vi "List Queues.vi"(6 "Name Prefix":string, 8 "error in (no error)":errorcluster, 9 "Region":T1, 11 "AWS Credentials":T2) -> (0 "error out":errorcluster, 3 "SQS Queues":refnum<class "Queue.lvclass">[](array[class]))   [LabVIEW 2015, in "NI_AWS_SQS.lvlib" / "Queue.lvclass"]
doc: "Returns a list of your queues. The maximum number of queues that can be returned is 1,000. If you specify a value for the optional QueueNamePrefix parameter, only queues with a name that begins with the specified value are returned."
uses:
  Queue.lvclass
  Core/HTTP Request/AWS Credentials.ctl
  Core/HTTP Request/Region.ctl
  Core/HTTP Request/Request Options.ctl
  Core/HTTP Request/Name Value Pair.ctl
  Core/HTTP Request/Region handling.ctl
  Core/HTTP Request/URL formatting.ctl
  Core/HTTP Request/HTTP Request.lvclass/HTTP Request.ctl
  Queue.lvclass/Queue.ctl
  Write Account Number.vi
  Write Name.vi
  Write URL.vi
  Core/HTTP Request/Write Credentials.vi
  Core/HTTP Request/Write Region.vi
  Core/HTTP Request/Write Service.vi
  Core/HTTP Request/Write Verify Server.vi
  Core/HTTP Request/HTTP Request.lvclass
  XML Parsing/NI_XML Parsing.lvlib
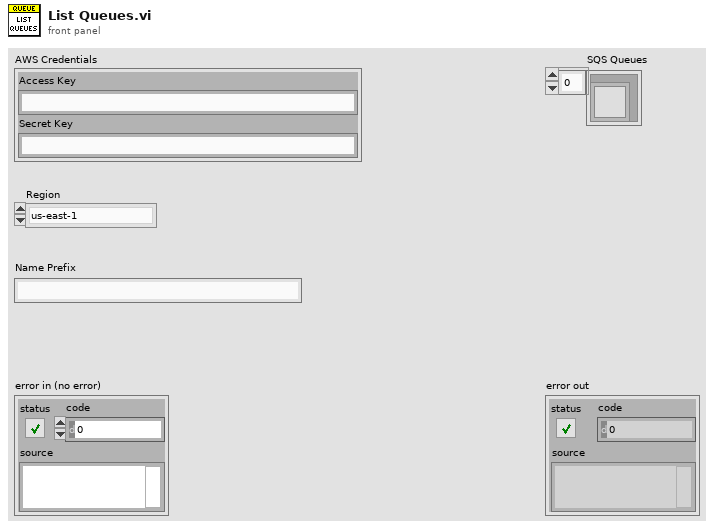
[diagram p1: front panel]
types:
  T1 = typedef "NI_AWS_Core.lvlib/HTTP Request.lvclass/Region.ctl" = enum16{"us-east-1", "us-east-2", "us-west-1", "us-west-2", "ap-northeast-1", "ap-northeast-2", "ap-southeast-1", "ap-southeast-2", "ca-central-1", "eu-central-1", "eu-west-1", "eu-west-2", "sa-east-1"}
  T2 = typedef "NI_AWS_Core.lvlib/HTTP Request.lvclass/AWS Credentials.ctl" = cluster{"Access Key":string, "Secret Key":string}
  T3 = typedef "NI_AWS_Core.lvlib/HTTP Request.lvclass/Name Value Pair.ctl" = cluster{"name":string, "value":string}
  T4 = typedef "NI_AWS_Core.lvlib/HTTP Request.lvclass/Request Options.ctl" = cluster{"request headers":T3[], "request parameters":T3[], "request body":string, "region handling":T5, "URL formatting":T6}
  T5 = typedef "NI_AWS_Core.lvlib/HTTP Request.lvclass/Region handling.ctl" = enum16{"use region everywhere", "use region (authentication only)", "use region (URL only)", "ignore region everwhere"}
  T6 = typedef "NI_AWS_Core.lvlib/HTTP Request.lvclass/URL formatting.ctl" = enum16{"region-", "region."}
  T7 = typedef "NI_AWS_Core.lvlib/HTTP Request.lvclass/Response.ctl" = cluster{"Headers":string, "Body":string}
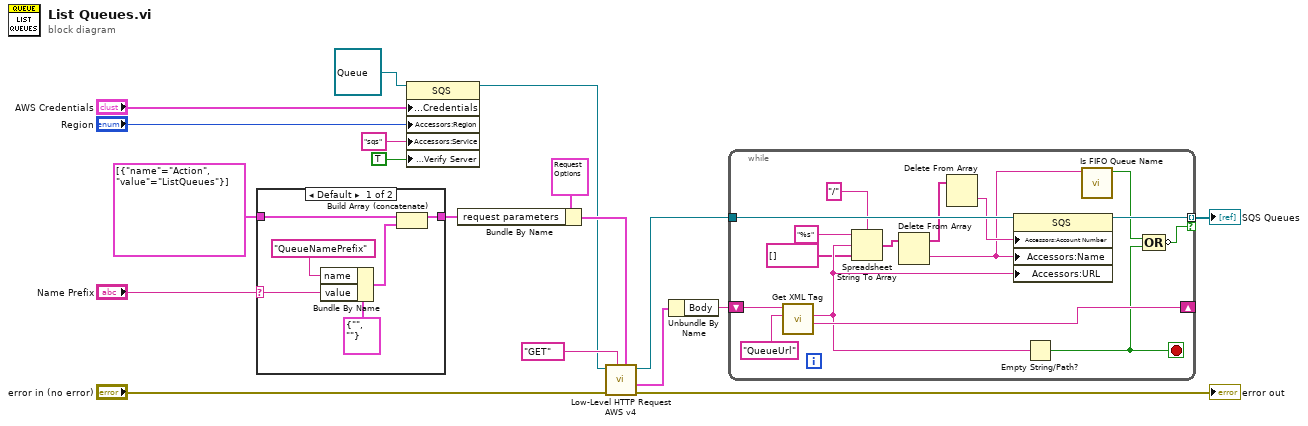
[diagram p0: block diagram]
diagram:
  n1 = case shown="Default" "Name Prefix" {
    selector: "Name Prefix" -> [w20 _]
    tunnel: T3[] [{"name"="Action", "value"="ListQueues"}] ("request parameters") -> [w24 w25]
    tunnel: [w23 w25] -> w10
    frame Default {
      n2 = Bundle By Name(cluster=T3 {"name"="", "value"=""} ("Cluster"), "name"="QueueNamePrefix", "value"=w20) -> (w21:T3)
      n3 = Build Array (concatenate)(w24, w21) -> (w23:T3[])
    }
    frame "" {
    }
  }
  n4 = property class="SQS"(reference=refnum<class "Queue.lvclass"> refnum ("NI_SQS.lvlib:SQS"), "Accessors:Credentials"="AWS Credentials", "Accessors:Region"="Region", "Accessors:Service"="sqs" ("Service"), "Accessors:Verify Server"=TRUE ("Verify Server")) -> (reference out=w1:refnum<class "Queue.lvclass">)  [unwired: 1 in, 1 out]
  n5 = Bundle By Name(cluster=T4 {"request headers"=[], "request parameters"=[{"name"="Action", "value"="ListQueues"}], "request body"="", "region handling"=enum."use region everywhere", "URL formatting"=enum."region."} ("Request Options"), "request parameters"=w10) -> (w2:T4)
  n6 = call "Low-Level HTTP Request AWS v4.vi"("Request Options"=w2, "HTTP-Verb"="GET", "error in (no error)"="error in (no error)", "AWS Core in"=w1) -> ("error out"=→"error out":errorcluster, "Response"=w5:T7, "AWS Core out"=w4:refnum<class "Queue.lvclass">)  [unwired: 4 in, 1 out]
  n7 = Unbundle By Name(w5) -> ("Body"=w7:string)
  n8 = while {
    shift-right: [w40] -> _
    shift-left: w7 -> [w41]
    tunnel: w4 -> [w38]
    tunnel: [w37] -> w6 mode=indexing if=w28
    stop <- w29 stop-if-true
    n9 = call "Get XML Tag.vi"("Tag name"="QueueUrl", "XML String in"=w41) -> ("Remaining string"=w40:string, "Tag value"=w36:string)  [unwired: 5 in, 3 out]
    n10 = Spreadsheet String To Array(delimiter (Tab)="/", format string="%s", spreadsheet string=w36, array type (2D Dbl)=string[] []) -> (array=w32:string[])
    n11 = Delete From Array(array=w32) -> (deleted portion=w27:string, array with subset deleted=w31:string[])  [unwired: 2 in]
    n12 = Delete From Array(array=w31) -> (deleted portion=w30:string)  [unwired: 2 in, 1 out]
    n13 = property class="SQS"(reference=w38, "Accessors:Account Number"=w30, "Accessors:Name"=w27, "Accessors:URL"=w36) -> (reference out=w37:refnum<class "Queue.lvclass">)  [unwired: 1 in, 1 out]
    n14 = Empty String/Path?(string/path=w36) -> (empty?=w29:bool)
    n15 = call "Is FIFO Queue Name.vi"("Name"=w27) -> ("FIFO Queue"=w26:bool)  [unwired: 10 in]
    n16 = Compound Arithmetic op=OR(w26, w29) -> (invert w28:bool)
  }
  "SQS Queues" <- w6
